vi "Track_Model.vi"(9 "Car_Speed":dbl, 10 "Theta_Steer":dbl, 11 "Sample_Time":dbl) -> (1 "car_pos_polar":cdb[](array[numeric]), 2 "car_pos":dbl[](array[numeric]), 3 "car_theta":dbl)   [LabVIEW 2018]
uses:
  <vilib>/Simulation/Implementation/Shared/SIMSCR Execution Mode.ctl
  <vilib>/Simulation/Scripting/Companion Diagram/SimConfigNode/SimParams.ctl
  <vilib>/Simulation/Scripting/Companion Diagram/SimConfigNode/_simSolvers.ctl
  <vilib>/Simulation/Param Hierarchy/Typedefs/SIMPH Param Control Actions.ctl
  <vilib>/Simulation/Implementation/Shared/NILVSim_ParamChanged.vi
  <vilib>/Simulation/Implementation/Shared/NILVSIM_BeginStep.vi
  <vilib>/Simulation/Utility/Implementation/NILVSim Memory.llb/NILVSim Memory (core).vi
  <vilib>/Simulation/Implementation/Shared/NILVSim_Manager.vi
  <vilib>/Utility/error.llb/Clear Errors.vi
  <vilib>/Simulation/Implementation/Shared/NILVSim_FinalizeModel.vi
  <vilib>/Simulation/Implementation/Shared/SIM Unbundle Sim Info.vi
  <vilib>/Simulation/Implementation/Shared/SIMSH Read Queue.vi
  <vilib>/Simulation/Implementation/Shared/NILVSim_Initialize.vi
  <vilib>/imath/engines/lvmath2/RunTimeEngine/BuiltInFunctions/atan2/NIMS_atan2.vi
  <instcachedir>/0/NIMS_atan2_A91AA4A7D42247EDBE8F76DB99AF04A4.lvgen/NIMS_atan2_A91AA4A7D42247EDBE8F76DB99AF04A4_001.vi
  <vilib>/imath/engines/lvmath2/RunTimeEngine/IndexReplace/NIMS V(S)=S.vi
  <instcachedir>/0/NIMS V(S)=S_420DA4522869420292A92FA3CC108C4E.lvgen/NIMS V(S)=S_420DA4522869420292A92FA3CC108C4E_000.vi
  <vilib>/imathl/engines/lvmath/Functions/Error Handling/Create Error.vi
  <instcachedir>/0/NIMS V(S)=S_420DA4522869420292A92FA3CC108C4E.lvgen/NIMS V(S)=S_420DA4522869420292A92FA3CC108C4E_001.vi
  <vilib>/imath/engines/lvmath2/RunTimeEngine/IndexRead/NIMS V(S).vi
  <instcachedir>/0/NIMS V(S)_0488751826AF41519A22953C041130DC.lvgen/NIMS V(S)_0488751826AF41519A22953C041130DC_000.vi
  <vilib>/imath/engines/lvmath2/RunTimeEngine/ErrorHandling/NIMS_Create Error From Enums.vi
  <instcachedir>/0/NIMS V(S)_0488751826AF41519A22953C041130DC.lvgen/NIMS V(S)_0488751826AF41519A22953C041130DC_003.vi
  <vilib>/imath/engines/lvmath2/RunTimeEngine/NodeEndStatement/NIMS_NodeEndStatement_Output.vi
  <instcachedir>/0/NIMS_NodeEndStatement_Output_53EC0D466D134D7ABD903AC30B43404B.lvgen/NIMS_NodeEndStatement_Output_53EC0D466D134D7ABD903AC30B43404B_005.vi
  <instcachedir>/0/NIMS_NodeEndStatement_Output_53EC0D466D134D7ABD903AC30B43404B.lvgen/NIMS_NodeEndStatement_Output_53EC0D466D134D7ABD903AC30B43404B_000.vi
  <instcachedir>/0/NIMS_NodeEndStatement_Output_53EC0D466D134D7ABD903AC30B43404B.lvgen/NIMS_NodeEndStatement_Output_53EC0D466D134D7ABD903AC30B43404B_001.vi
  <vilib>/imath/engines/lvmath2/RunTimeEngine/ErrorHandling/NIMS_Finalize Error.vi
  <vilib>/Simulation/Utility/Implementation/NILVSim Get Time and IsAcceptedStep.vi
  <vilib>/Simulation/Implementation/Shared/NILVSim_GetModelError.vi
  <vilib>/Simulation/Implementation/Shared/SIM SimErrorHandler.vi
  <vilib>/Simulation/Implementation/Shared/SIM Bundle Sim Info.vi
  <vilib>/Simulation/Scripting/Companion Diagram/SimConfigNode/SimDog.xnode
  <vilib>/Simulation/Implementation/XNodeFramework/SimXNode/SimX.xnode
  <vilib>/Simulation/Implementation/Shared/NI_SIM_Implementation.lvlib
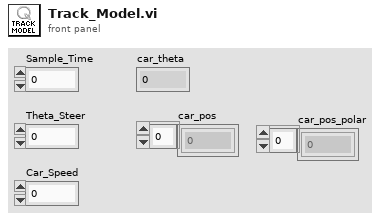
[diagram p1: front panel]
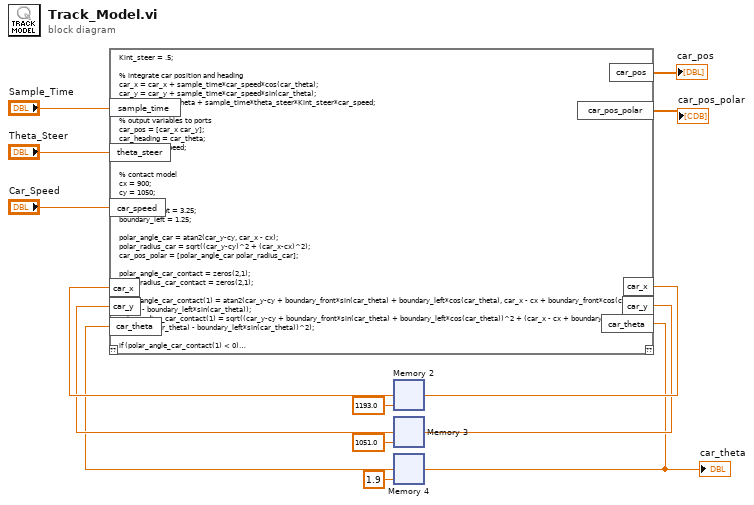
[diagram p0: block diagram]
diagram:
  n1 = mathscript code="Kint_steer = .5;\n\n% integrate car position and heading\ncar_x = car_x + sample_time*car_speed*cos(car_theta);\ncar_y = car_y + sample_time*car_speed*sin(car_theta);\ncar_theta = car_theta + sample_time*theta_steer*Kint_steer*car_speed;\n\n% output variables to ports\ncar_pos = [car_x car_y];\ncar_heading = car_theta;\nspeed = car_speed;\n\n\n% contact model\ncx = 900;\ncy = 1050;\n\nboundary_front = 3.25;\nboundary_left = 1.25; \n\npolar_angle_car = atan2(car_y-cy, car_x - cx);\npolar_radius_car = sqrt((car_y-cy)^2 + (car_x-cx)^2);\ncar_pos_polar = [polar_angle_car polar_radius_car];\n\npolar_angle_car_contact = zeros(2,1);\npolar_radius_car_contact = zeros(2,1);\n\npolar_angle_car_contact(1) = atan2(car_y-cy + boundary_front*sin(car_theta) + boundary_left*cos(car_theta), car_x - cx + boundary_front*cos(car_theta) - boundary_left*sin(car_theta));\npolar_radius_car_contact(1) = sqrt((car_y-cy + boundary_front*sin(car_theta) + boundary_left*cos(car_theta))^2 + (car_x - cx + boundary_front*cos(car_theta) - boundary_left*sin(car_theta))^2);\n\nif (polar_angle_car_contact(1) < 0)\n    polar_angle_car_contact(1) = polar_angle_car_contact(1) + 2*pi;\nend\n\npolar_angle_car_contact(2) = atan2(car_y-cy + boundary_front*sin(car_theta) - boundary_left*cos(car_theta), car_x - cx + boundary_front*cos(car_theta) + boundary_left*sin(car_theta));\npolar_radius_car_contact(2) = sqrt((car_y-cy + boundary_front*sin(car_theta) - boundary_left*cos(car_theta))^2 + (car_x - cx + boundary_front*cos(car_theta) + boundary_left*sin(car_theta))^2);\n\nif (polar_angle_car_contact(2) < 0)\n    polar_angle_car_contact(2) = polar_angle_car_contact(2) + 2*pi;\nend\n\n%% copied from barrier model\n\ntheta = polar_angle_car_contact(1);\n\nFr = (200 + 100*sin(-2*theta));\nx_inner = Fr*cos(theta);\ny_inner = Fr*sin(theta);\n\n\ntheta = polar_angle_car_contact(2);\n\nFr = (400 + 100*sin(-2*theta)  );\nx_outer = Fr*cos(theta);\ny_outer = Fr*sin(theta);\n\n\nif (polar_radius_car_contact(1) < sqrt(x_inner^2 + y_inner^2) || ...\n    polar_radius_car_contact(1) > sqrt(x_outer^2 + y_outer^2) )\n    \n    car_theta = car_theta - 0.1;\n\nelseif (polar_radius_car_contact(2) < sqrt(x_inner^2 + y_inner^2) || ...\n    polar_radius_car_contact(2) > sqrt(x_outer^2 + y_outer^2) )\n\n    car_theta = car_theta + 0.1;\nend"("car_x"=w7, "car_y"=w6, "car_theta"=w5, "sample_time"="Sample_Time", "theta_steer"="Theta_Steer", "car_speed"="Car_Speed") -> ("car_x"=w10:dbl, "car_y"=w9:dbl, "car_theta"=w8:dbl, "car_pos_polar"=→"car_pos_polar":cdb[], "car_pos"=→"car_pos":dbl[])  [unwired: 1 in, 1 out]
  "car_theta" <- w8
  n2 = xnode ("Memory 2")("input"=w10, "initial value"=1193.0 ("initial value 2")) -> ("output"=w7:dbl)  [unwired: 4 in]
  n3 = xnode ("Memory 3")("input"=w9, "initial value"=1051.0 ("initial value 3")) -> ("output"=w6:dbl)  [unwired: 4 in]
  n4 = xnode ("Memory 4")("input"=w8, "initial value"=1.9) -> ("output"=w5:dbl)  [unwired: 4 in]
